vi "Set_Step.vi"(8 "error in (no error)":errorcluster, 10 "Set_stepcount":i32, 11 "Lifter_motor in":refnum<class "Lifter_motor.lvclass">) -> (0 "error out":errorcluster, 3 "Lifter_motor out":refnum<class "Lifter_motor.lvclass">)   [LabVIEW 2019, in "Lifter_motor.lvclass"]
uses:
  Lifter_motor.lvclass
  Lifter_motor.lvclass/Lifter_motor.ctl
  TCP Class/LifterTCP.lvclass
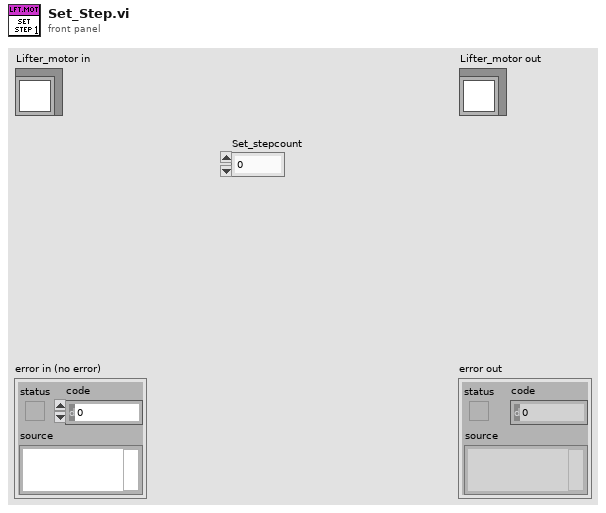
[diagram p1: front panel]
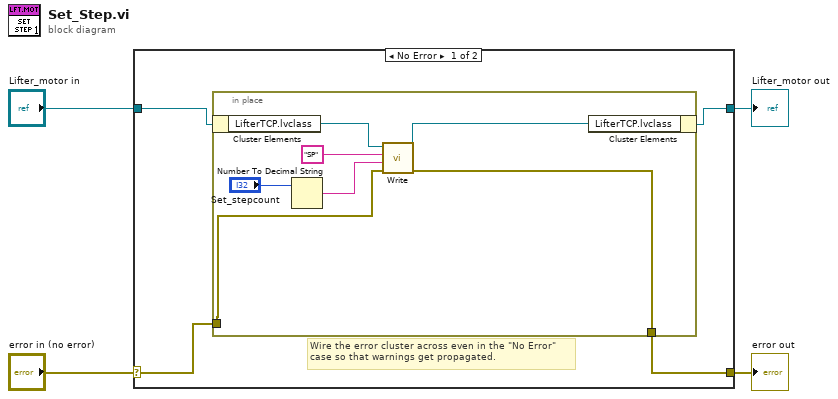
[diagram p0: block diagram]
diagram:
  n1 = case shown="No Error" "error in (no error)" {
    selector: "error in (no error)" -> [w6 w17]
    tunnel: [w5 w17] -> w3
    tunnel: [w7 w16] -> w1
    tunnel: "Lifter_motor in" -> [w8 w16]
    frame No Error {
      # "Wire the error cluster across even in the \"No Error\"\ncase so that warnings get propagated."
      n2 = in-place {
        in-place-border: w6 -> [w12]
        in-place-border: [w11] -> w5
        n3 = in-place-cluster #1(w8) -> ("LifterTCP.lvclass"=w15:refnum<class "LifterTCP.lvclass">)
        n4 = Number To Decimal String(number="Set_stepcount") -> (decimal integer string=w9:string)  [unwired: 1 in]
        n5 = call "Write.vi"("error in (no error)"=w12, "Parameter 2"=w9, "Parameter 1"="SP", "LifterTCP in"=w15) -> ("error out"=w11:errorcluster, "LifterTCP out"=w14:refnum<class "LifterTCP.lvclass">)  [unwired: 5 in, 1 out]
        n6 = in-place-cluster #1("LifterTCP.lvclass"=w14) -> (w7:refnum<class "Lifter_motor.lvclass">)
      }
    }
    frame Error {
    }
  }
  "error out" <- w3
  "Lifter_motor out" <- w1
